vi "Path Keeper_Check If Valid.vi"(8 "error In":errorcluster, 9 "File(f)\nDirectory(t) In":bool, 11 "path In":path) -> (0 "error Out":errorcluster, 3 "Valid Out":bool)   [LabVIEW 2015]
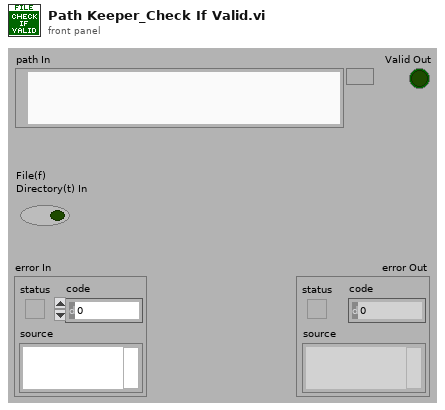
[diagram p1: front panel]
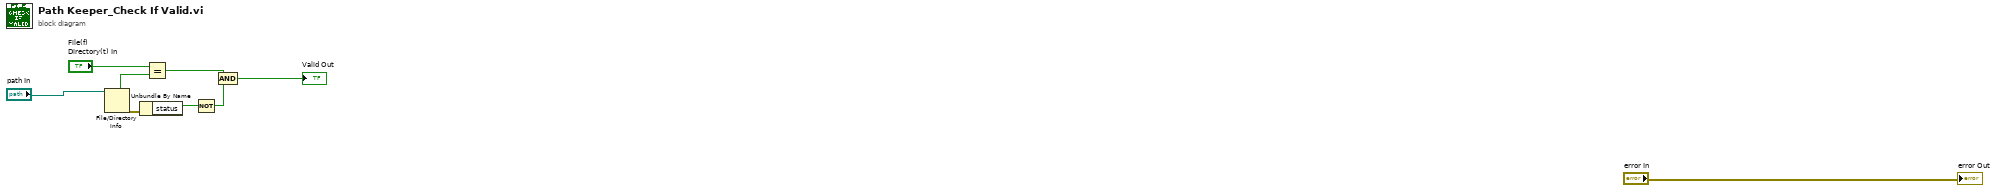
[diagram p0: block diagram]
diagram:
  n1 = File/Directory Info(path="path In") -> (directory=w4:bool, error out=w3:errorcluster)  [unwired: 1 in, 5 out]
  n2 = Unbundle By Name(w3) -> ("status"=w6:bool)
  n3 = Equal?(x="File(f)\nDirectory(t) In", y=w4) -> (x = y?=w8:bool)
  n4 = Not(x=w6) -> (.not. x?=w7:bool)
  n5 = And(x=w8, y=w7) -> (x .and. y?=→"Valid Out":bool)
  "error Out" <- "error In"
